vi "Save to File.vi"(8 "error in (no error)":errorcluster, 10 "Path":path, 11 "GPack File in":refnum<class "GPack File.lvclass">) -> (0 "error out":errorcluster, 3 "GPack File out":refnum<class "GPack File.lvclass">)   [LabVIEW 2020, in "GPack.lvlib" / "GPack File.lvclass"]
uses:
  GPack File.lvclass
  File Contents.ctl
  Package Info.ctl
  Dependency.ctl
  GPack File.lvclass/GPack File.ctl
  fb048cc8-f45a-4637-bd27-992e99e90cdf.vi
  <vilib>/JDP Science/JSONtext/Variant to JSON Text.vi
  <vilib>/JDP Science/JSONtext/LVClass Serializer/JSONtext LVClass Serializer.lvclass
  GPack.lvlib
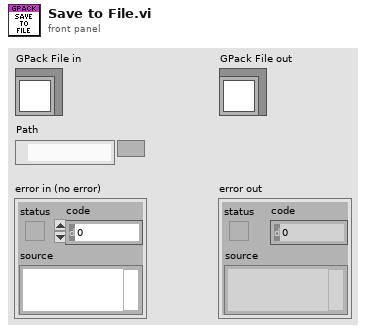
[diagram p1: front panel]
types:
  T1 = typedef "GPack.lvlib/GPack File.lvclass/File Contents.ctl" = cluster{"Info":T2, "Dependencies":T3[]}
  T2 = typedef "GPack.lvlib/Package Info.ctl" = cluster{"Name":string, "Type":string, "Host":string, "Path":string, "Branch":string, "Version":string, "License":string}
  T3 = typedef "GPack.lvlib/Dependency.ctl" = cluster{"Info":T2, "Path":path}
  T4 = enum16{"open", "replace", "create", "open or create", "replace or create", "replace or create with confirmation"}
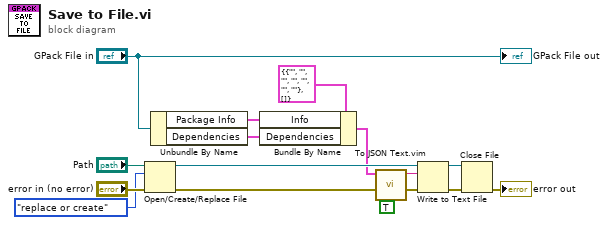
[diagram p0: block diagram]
diagram:
  n1 = Open/Create/Replace File(file path (use dialog)="Path", error in="error in (no error)", operation (0:open)=T4."replace or create") -> (refnum out=w7:refnum<file>, error out=w15:errorcluster)  [unwired: 3 in, 1 out]
  n2 = Unbundle By Name("GPack File in") -> ("Package Info"=w9:T2, "Dependencies"=w8:T3[])
  n3 = Bundle By Name(cluster=T1 {"Info"={"Name"="", "Type"="", "Host"="", "Path"="", "Branch"="", "Version"="", "License"=""}, "Dependencies"=[]} ("File Contents"), "Info"=w9, "Dependencies"=w8) -> (w3:T1)
  n4 = call "To JSON Text.vim"("Pretty Print?"=TRUE, "error in (no error)"=w15, "Anything"=w3) -> ("error out"=w16:errorcluster, "<JSON>"=w2:string)  [unwired: 7 in]
  n5 = Write to Text File(file (use dialog)=w7, text=w2, error in=w16) -> (refnum out=w5:refnum<file>, error out=w6:errorcluster)  [unwired: 1 in, 1 out]
  n6 = Close File(refnum=w5, error in=w6) -> (error out=→"error out":errorcluster)  [unwired: 1 out]
  "GPack File out" <- "GPack File in"
